vi "StopChannel.vi"(8 "error in (no error)":errorcluster, 10 "Channel":u8, 11 "ID In":i32) -> (0 "error out":errorcluster, 3 "ID Out":i32)   [LabVIEW 2022 SP3, in "EClib functions.lvlib"]
doc: "This VI stops loaded ecc protocols on the selected channel."
uses:
  EClib functions.lvlib
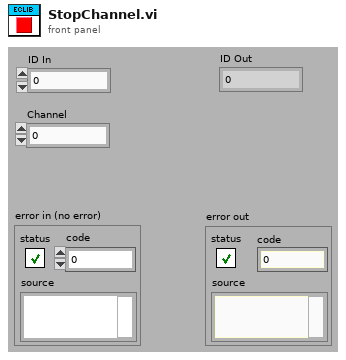
[diagram p1: front panel]
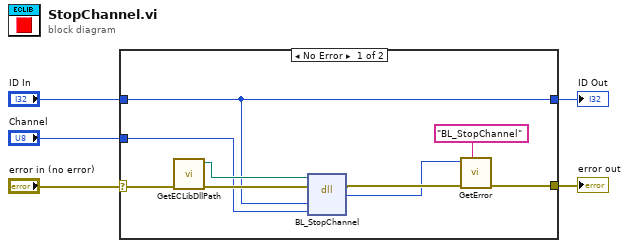
[diagram p0: block diagram]
diagram:
  n1 = case shown="No Error" "error in (no error)" {
    selector: "error in (no error)" -> [w12 w15]
    tunnel: [w13 w15] -> w5
    tunnel: "ID In" -> [w6 _]
    tunnel: "Channel" -> [w9 _]
    tunnel: [w6 _] -> w1
    frame No Error {
      n2 = call "GetECLibDllPath.vi"("error in (no error)"=w12) -> ("error out"=w11:errorcluster, "ECLibDLLPath"=w14:path)  [unwired: 9 in]
      n3 = dll-call lib="?" fn="BL_StopChannel"(path in=w14, error in=w11, "arg1"=w6, "arg2"=w9) -> (error out=w10:errorcluster, "return type"=w7:i32)  [unwired: 3 in, 1 out]
      n4 = call "GetError.vi"("DLLFunction"="BL_StopChannel", "error in"=w10, "code"=w7) -> ("error out"=w13:errorcluster)  [unwired: 8 in]
    }
    frame Error {
    }
  }
  "error out" <- w5
  "ID Out" <- w1
